vi "Module Init.vi"(8 "error in (no error)":errorcluster, 11 "Triggered Logger in":refnum<class "Triggered Logger.lvclass">) -> (0 "error out":errorcluster, 3 "Triggered Logger out":refnum<class "Triggered Logger.lvclass">)   [LabVIEW 2020, in "VolatusData.lvlib" / "Triggered Logger.lvclass"]
uses:
  Triggered Logger.lvclass
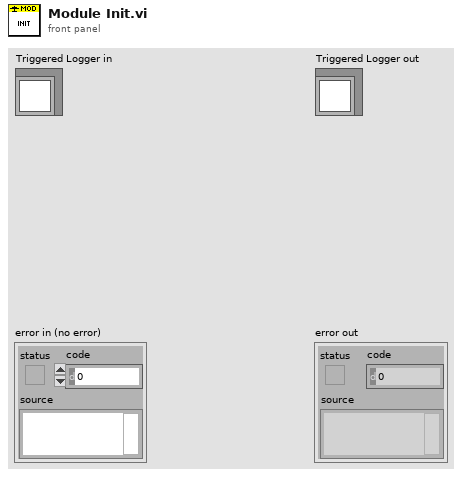
[diagram p1: front panel]
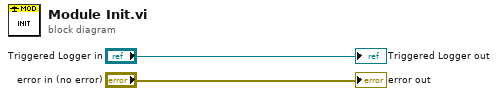
[diagram p0: block diagram]
diagram:
  "error out" <- "error in (no error)"
  "Triggered Logger out" <- "Triggered Logger in"
